vi "Simulation-03.vi"() -> (0 "lib error out":errorcluster, 3 "success":bool)   [LabVIEW 2020]
uses:
  librarian_class/typedefs/book_state--enum.ctl
  shared/request--enum.ctl
  librarian_class/librarian.lvclass
  client_class/client.lvclass
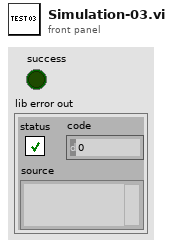
[diagram p1: front panel]
types:
  T1 = typedef "request--enum.ctl" = enum16{"CHECKIN", "CHECKOUT"}
  T2 = typedef "librarian.lvclass/book_state--enum.ctl" = enum16{"CHECKEDIN", "CHECKEDOUT", "DAMAGED"}
  T3 = typedef "message--cluster.ctl" = cluster{"header":string, "cmd":T1, "title":string, "book":string}
  T4 = typedef "librarian.lvclass/lib_map_value--cluster.ctl" = cluster{"book state":T2, "text":string, "hash":string}
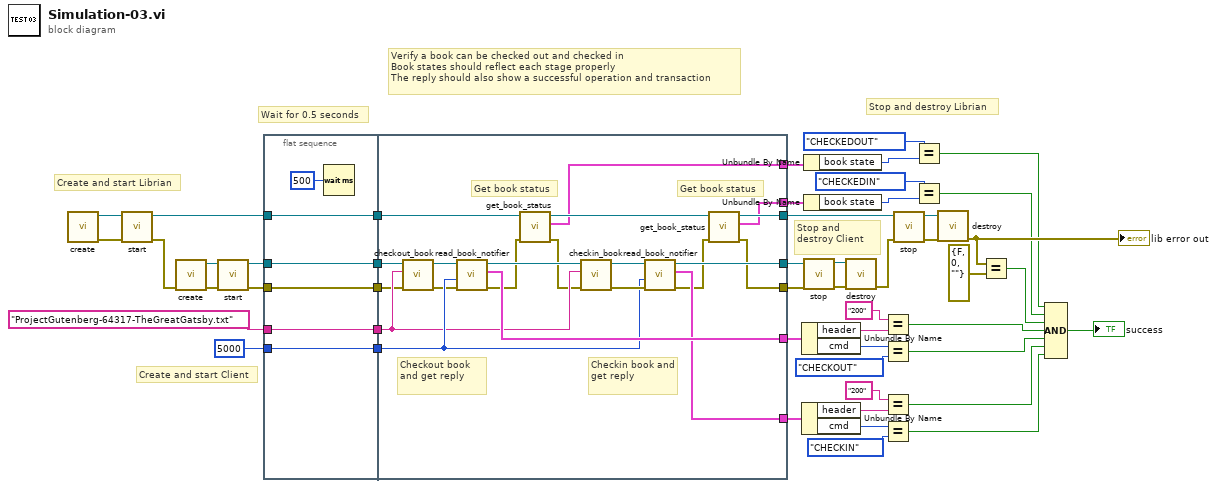
[diagram p0: block diagram]
diagram:
  # "Verify a book can be checked out and checked in\nBook states should reflect each stage properly\nThe reply should also show a successful operation and transaction"
  # "Stop and destroy Client"
  # "Wait for 0.5 seconds"
  # "Create and start Client"
  # "Stop and destroy Librian"
  # "Create and start Librian"
  n1 = call "create.vi"() -> ("error out"=w48:errorcluster, "librarian_sm out"=w49:refnum<class "librarian.lvclass">)  [unwired: 10 in]
  n2 = call "start.vi"("error in (no error)"=w48, "librarian_sm in"=w49) -> ("error out"=w28:errorcluster, "librarian_sm out"=w39:refnum<class "librarian.lvclass">)  [unwired: 8 in]
  n3 = call "create.vi"("error in (no error)"=w28) -> ("error out"=w44:errorcluster, "librarian_sm out"=w45:refnum<class "client.lvclass">)  [unwired: 9 in]
  n4 = call "start.vi"("error in (no error)"=w44, "librarian_sm in"=w45) -> ("error out"=w41:errorcluster, "librarian_sm out"=w40:refnum<class "client.lvclass">)  [unwired: 8 in]
  n5 = flat-sequence {
    tunnel: "ProjectGutenberg-64317-TheGreatGatsby.txt" ("book title") -> [w50]
    tunnel: 5000 ("timeout in ms (-1)") -> [w53]
    tunnel: w39 -> [w54]
    tunnel: w40 -> [w55]
    tunnel: w41 -> [w51]
    tunnel: [w51] -> w33
    tunnel: [w55] -> w32
    tunnel: [w54] -> w31
    tunnel: [w53] -> w30
    tunnel: [w50] -> w29
    tunnel: [w76] -> w18
    tunnel: [w60] -> w36
    tunnel: [w70] -> w37
    tunnel: [w58] -> w38
    tunnel: [w69] -> w9
    tunnel: w29 -> [w71]
    tunnel: w30 -> [w72]
    tunnel: w31 -> [w64]
    tunnel: w32 -> [w67]
    tunnel: w33 -> [w68]
    tunnel: [w57] -> w21
    tunnel: [w56] -> w26
    frame #0 {
      n6 = Wait (ms)(milliseconds to wait=u32 500) -> ()  [unwired: 1 out]
    }
    frame #1 {
      # "Get book status"
      # "Get book status"
      # "Checkin book and get reply"
      # "Checkout book and get reply"
      n7 = call "checkout_book.vi"("error in (no error)"=w68, "book title"=w71, "client in"=w67) -> ("error out"=w65:errorcluster, "client out"=w66:refnum<class "client.lvclass">)  [unwired: 7 in]
      n8 = call "read_book_notifier.vi"("error in (no error)"=w65, "timeout in ms (-1)"=w72, "client in"=w66) -> ("error out"=w63:errorcluster, "msg"=w76:T3, "client out"=w75:refnum<class "client.lvclass">)  [unwired: 6 in]
      n9 = call "get_book_status.vi"("error in (no error)"=w63, "librarian in"=w64) -> ("error out"=w62:errorcluster, "book status"=w56:T4, "librarian out"=w59:refnum<class "librarian.lvclass">)  [unwired: 7 in]
      n10 = call "checkin_book.vi"("error in (no error)"=w62, "book title"=w71, "client in"=w75) -> ("error out"=w73:errorcluster, "client out"=w74:refnum<class "client.lvclass">)  [unwired: 7 in]
      n11 = call "read_book_notifier.vi"("error in (no error)"=w73, "timeout in ms (-1)"=w72, "client in"=w74) -> ("error out"=w61:errorcluster, "msg"=w69:T3, "client out"=w70:refnum<class "client.lvclass">)  [unwired: 6 in]
      n12 = call "get_book_status.vi"("error in (no error)"=w61, "librarian in"=w59) -> ("error out"=w60:errorcluster, "book status"=w57:T4, "librarian out"=w58:refnum<class "librarian.lvclass">)  [unwired: 7 in]
    }
  }
  n13 = Unbundle By Name(w18) -> ("header"=w17:string, "cmd"=w15:T1)
  n14 = Unbundle By Name(w9) -> ("header"=w10:string, "cmd"=w12:T1)
  n15 = Unbundle By Name(w26) -> ("book state"=w25:T2)
  n16 = Unbundle By Name(w21) -> ("book state"=w22:T2)
  n17 = call "stop.vi"("error in (no error)"=w36, "librarian_sm in"=w37) -> ("error out"=w42:errorcluster, "librarian_sm out"=w43:refnum<class "client.lvclass">)  [unwired: 8 in]
  n18 = call "destroy.vi"("error in (no error)"=w42, "librarian_sm in"=w43) -> ("error out"=w27:errorcluster)  [unwired: 8 in, 1 out]
  n19 = Equal?(x="200", y=w17) -> (x = y?=w5:bool)
  n20 = Equal?(x=w15, y=request--enum."CHECKOUT") -> (x = y?=w4:bool)
  n21 = Equal?(x="200", y=w10) -> (x = y?=w3:bool)
  n22 = Equal?(x=w12, y=request--enum."CHECKIN") -> (x = y?=w2:bool)
  n23 = call "stop.vi"("error in (no error)"=w27, "librarian_sm in"=w38) -> ("error out"=w46:errorcluster, "librarian_sm out"=w47:refnum<class "librarian.lvclass">)  [unwired: 8 in]
  n24 = Equal?(x=book_state--enum."CHECKEDOUT", y=w25) -> (x = y?=w8:bool)
  n25 = Equal?(x=book_state--enum."CHECKEDIN", y=w22) -> (x = y?=w7:bool)
  n26 = call "destroy.vi"("error in (no error)"=w46, "librarian_sm in"=w47) -> ("error out"=w20:errorcluster)  [unwired: 8 in, 1 out]
  "lib error out" <- w20
  n27 = Equal?(x=w20, y=errorcluster {"status"=FALSE, "code"=0, "source"=""}) -> (x = y?=w6:bool)
  n28 = Compound Arithmetic op=AND(w8, w7, w6, w5, w4, w3, w2) -> (→"success":bool)
